vi "main_array.vi"() -> ()   [LabVIEW 2017]
uses:
  Bundle_array.ctl
panel:
  in  "stop":bool
  in  "Mode":enum32{"LIDAR", "Range detector"}(tab)
  out "Polar Plot":picture
  in  "Plot Color":u32(colorbox)=16715776
  in  "Grid Color":u32(colorbox)
  in  "Visible Section":u16(ring)=8
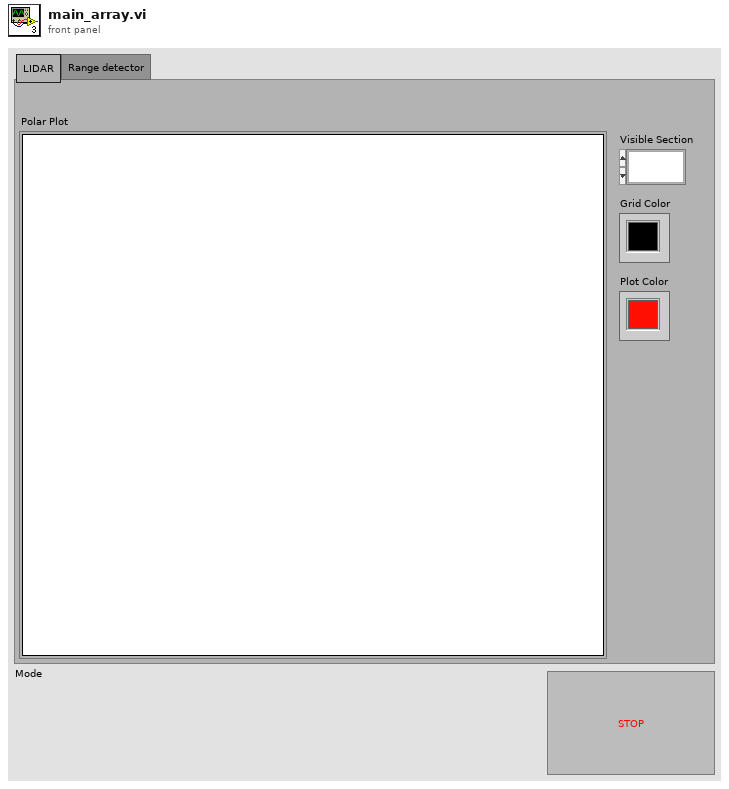
[diagram p1: front panel]
types:
  T1 = cluster{"maximum":dbl, "minimum":dbl, "clip to min":bool, "log?(F)":bool, "grid color":u32, "plot color":u32, "format and precision":cluster{"format":enum8{"Decimal", "Scientific", "Engineering", "Binary", "Octal", "Hex"}, "precision":u8}, "visible section":u16}
  T2 = typedef "LVBoundsTypeDef.ctl" = cluster{"Width":u32, "Height":u32}
  T3 = typedef "Bundle_array.ctl" = cluster{"Numeric":dbl, dbl}[]
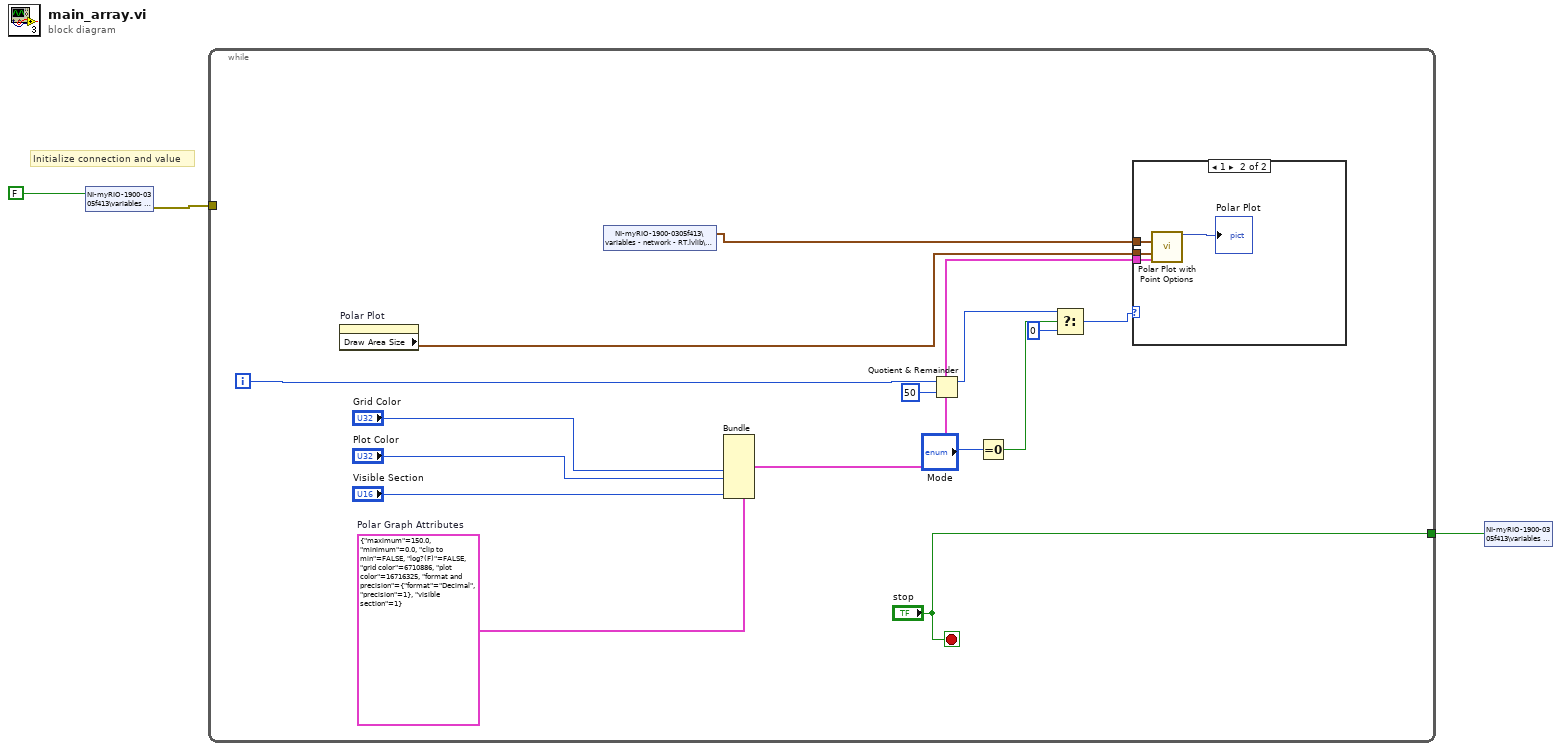
[diagram p0: block diagram]
diagram:
  # "Initialize connection and value"
  n1 = shared-variable "NI-myRIO-1900-0305f413\\variables - network - RT.lvlib\\stop"(FALSE) -> (error out=w2:errorcluster)  [unwired: 1 in]
  n2 = while {
    tunnel: ["stop"] -> w3
    tunnel: w2 -> [_]
    i -> [w10]
    stop <- "stop" stop-if-true
    w16 = T1 {"maximum"=150.0, "minimum"=0.0, "clip to min"=FALSE, "log?(F)"=FALSE, "grid color"=6710886, "plot color"=16716325, "format and precision"={"format"=enum."Decimal", "precision"=1}, "visible section"=1}  # Polar Graph Attributes
    n3 = property on="Polar Plot" class="Pict"() -> ("Draw Area Size"=w17:T2)  [unwired: 2 in, 2 out]
    n4 = shared-variable "NI-myRIO-1900-0305f413\\variables - network - RT.lvlib\\Bundle_array"() -> (w4:T3)  [unwired: 1 in, 1 out]
    n5 = Bundle(cluster=w16, "grid color"="Grid Color", "plot color"="Plot Color", "visible section"="Visible Section") -> (w12:T1)  [unwired: 5 in]
    n6 = Quotient & Remainder(x=w10, y=50) -> (x-y*floor(x/y)=w9:i32)  [unwired: 1 out]
    n7 = Equal To 0?(x="Mode") -> (x = 0?=w6:bool)
    n8 = Select(t=w9, s=w6, f=0) -> (s? t:f=w8:i32)
    n9 = case shown="1" w8 {
      tunnel: w17 -> [_ w22]
      tunnel: w4 -> [_ w20]
      tunnel: w12 -> [_ w19]
      frame 0, Default {
      }
      frame 1 {
        n10 = call <vilib>:"Polar Plot with Point Options.vi"("data array [mag, phase (deg)]"=w20, "dimensions (w,h)"=w22, "polar attributes"=w19) -> ("new picture"=→"Polar Plot":picture)  [unwired: 12 in]
      }
    }
  }
  n11 = shared-variable "NI-myRIO-1900-0305f413\\variables - network - RT.lvlib\\stop"(w3) -> ()  [unwired: 1 in, 1 out]
